vi "Get color.vi"(8 "Background color":T1(ring), 10 "Get color":T1(ring)) -> (0 "Colors cluster":cluster{u32, u32}[](array[cluster]), 2 "Color":u32(colorbox))   [LabVIEW 2020]
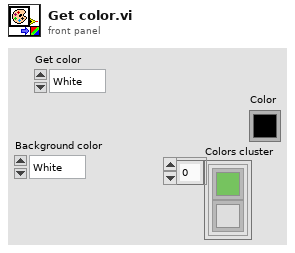
[diagram p1: front panel]
types:
  T1 = enum16{"White", "Black", "Green", "Blue", "Red", "Yellow", ""}
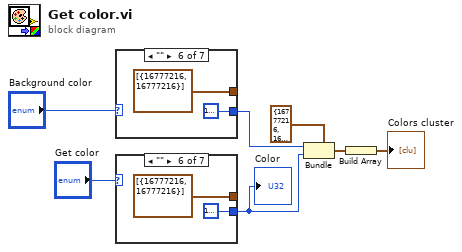
[diagram p0: block diagram]
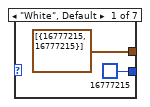
[diagram p2: hidden frame]
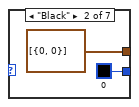
[diagram p3: hidden frame]
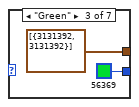
[diagram p4: hidden frame]
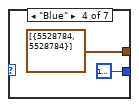
[diagram p5: hidden frame]
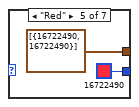
[diagram p6: hidden frame]
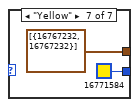
[diagram p7: hidden frame]
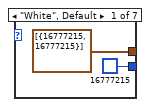
[diagram p8: hidden frame]
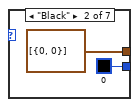
[diagram p9: hidden frame]
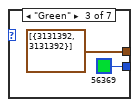
[diagram p10: hidden frame]
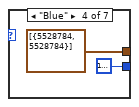
[diagram p11: hidden frame]
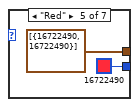
[diagram p12: hidden frame]
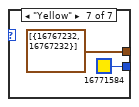
[diagram p13: hidden frame]
diagram:
  n1 = case shown="\"\"" "Background color" {
    tunnel: [u32 16777215 u32 0 u32 56369 u32 16777224 u32 16722490 u32 16777216 u32 16771584] -> w2
    tunnel: [cluster{u32, u32}[] [{16777215, 16777215}] ("Colors [4]") cluster{u32, u32}[] [{0, 0}] ("Colors [4]") cluster{u32, u32}[] [{3131392, 3131392}] ("Colors [4]") cluster{u32, u32}[] [{5528784, 5528784}] ("Colors [4]") cluster{u32, u32}[] [{16722490, 16722490}] ("Colors [4]") cluster{u32, u32}[] [{16777216, 16777216}] ("Colors [4]") cluster{u32, u32}[] [{16767232, 16767232}] ("Colors [4]")] -> _
    frame "White", Default {
    }
    frame "Black" {
    }
    frame "Green" {
    }
    frame "Blue" {
    }
    frame "Red" {
    }
    frame "" {
    }
    frame "Yellow" {
    }
  }
  n2 = case shown="\"\"" "Get color" {
    tunnel: [u32 16777215 u32 0 u32 56369 u32 16777224 u32 16722490 u32 16777216 u32 16771584] -> w1
    tunnel: [cluster{u32, u32}[] [{16777215, 16777215}] ("Colors [4]") cluster{u32, u32}[] [{0, 0}] ("Colors [4]") cluster{u32, u32}[] [{3131392, 3131392}] ("Colors [4]") cluster{u32, u32}[] [{5528784, 5528784}] ("Colors [4]") cluster{u32, u32}[] [{16722490, 16722490}] ("Colors [4]") cluster{u32, u32}[] [{16777216, 16777216}] ("Colors [4]") cluster{u32, u32}[] [{16767232, 16767232}] ("Colors [4]")] -> _
    frame "White", Default {
    }
    frame "Black" {
    }
    frame "Green" {
    }
    frame "Blue" {
    }
    frame "Red" {
    }
    frame "" {
    }
    frame "Yellow" {
    }
  }
  "Color" <- w1
  n3 = Bundle(cluster=cluster{u32, u32} {16777216, 16777216}, w2, w1) -> (w4:cluster{u32, u32})
  n4 = Build Array(w4) -> (→"Colors cluster":cluster{u32, u32}[])
